vi "Destroy User Define Events.vi"(8 "error in (no error)":errorcluster, 11 "CS++SeqEditor in":refnum<class "CS++SeqEditor.lvclass">) -> (0 "error out":errorcluster, 3 "CS++SeqEditor out":refnum<class "CS++SeqEditor.lvclass">)   [LabVIEW 2016, in "CS++SeqEditor.lvlib" / "CS++SeqEditor.lvclass"]
doc: "Destroy all user defined events."
uses:
  CS++SeqEditor.lvclass
  CS++SeqEditor.lvclass/CS++SeqEditor.ctl
  CSPP_Core/Actors/CS++GUIActor/CS++GUIActor.lvclass
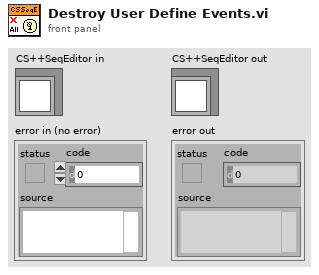
[diagram p1: front panel]
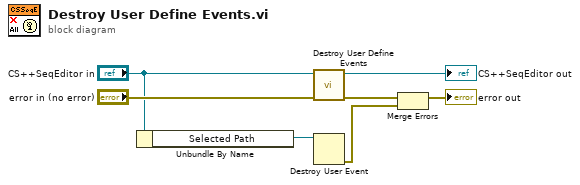
[diagram p0: block diagram]
diagram:
  n1 = Unbundle By Name("CS++SeqEditor in") -> ("Selected Path"=w3:refnum<user-event>)
  n2 = call-parent "Destroy User Define Events.vi"("error in (no error)"="error in (no error)", "CS++GUIActor in"="CS++SeqEditor in") -> ("error out"=w7:errorcluster, "CS++GUIActor out"=→"CS++SeqEditor out":refnum<class "CS++SeqEditor.lvclass">)  [unwired: 8 in]
  n3 = Destroy User Event(user event=w3) -> (error out=w1:errorcluster)  [unwired: 1 in]
  n4 = Merge Errors(w7, w1) -> (→"error out":errorcluster)
